vi "Init Abort Bearer.vi"(8 "error in (no error)":errorcluster, 11 "Guardian in":refnum<class "Guardian.lvclass">) -> (0 "error out":errorcluster, 3 "Guardian out":refnum<class "Guardian.lvclass">)   [LabVIEW 2026, in "TALOS.lvlib" / "Guardian.lvlib" / "Guardian.lvclass"]
uses:
  Guardian.lvclass
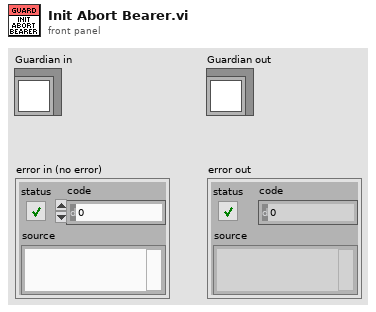
[diagram p1: front panel]
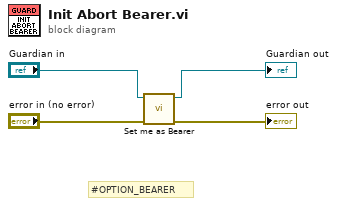
[diagram p0: block diagram]
diagram:
  # "#OPTION_BEARER"
  n1 = call "Set me as Bearer.vi"("error in"="error in (no error)", "Guardian in"="Guardian in") -> ("error out"=→"error out":errorcluster, "Guardian out"=→"Guardian out":refnum<class "Guardian.lvclass">)  [unwired: 8 in]
